vi "Modbus open serial port.vi"(11 "VISA resource name":refnum<visa-resource-name>) -> (0 "Error out":errorcluster, 3 "VISA resource name out":refnum<visa-resource-name>)   [LabVIEW 2020]
doc: "Modbus RTU for Invertek drives. Paul Nathan 18-JUN-2022."
uses:
  <vilib>/Instr/_visa.llb/VISA Open Access Mode.ctl
  Globals/Invertek Drive Params.vi
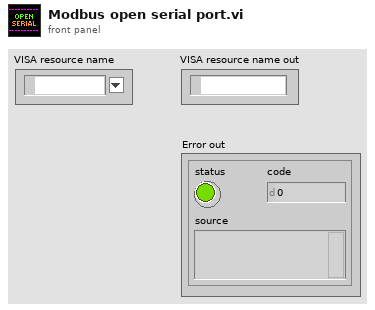
[diagram p1: front panel]
types:
  T1 = typedef "VISA Open Access Mode.ctl" = u32
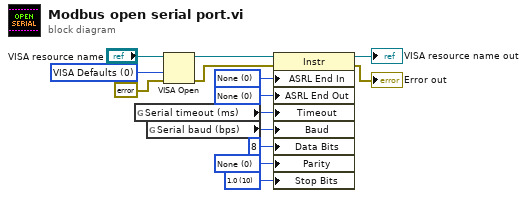
[diagram p0: block diagram]
diagram:
  w3 = u16 10 items=["1.0"=10, "1.5"=15, "2.0"=20] ("Serial Settings:Stop Bits")
  w4 = u16 0 items=["None", "Odd", "Even", "Mark", "Space"] ("Serial Settings:Parity")
  w6 = u16 0 items=["None", "Last Bit", "TermChar", "Break"] ("Serial Settings:End Mode for Writes")
  w11 = u16 0 items=["None", "Last Bit", "TermChar"] ("Serial Settings:End Mode for Reads")
  w14 = T1 0 items=["VISA Defaults"=0, "Exclusive Lock"=1, "Load Configured Settings"=4] ("Access Mode")
  n1 = global read "Invertek Drive Params.vi" "Serial timeout (ms)"() -> (w1:u32)
  n2 = global read "Invertek Drive Params.vi" "Serial baud (bps)"() -> (w2:u32)
  n3 = VISA Open(access mode=w14, error in (no error)=errorcluster {"status"=FALSE, "code"=0, "source"=""}, VISA resource name="VISA resource name") -> (VISA resource name=w8:refnum<visa-resource-name>, error out=w7:errorcluster)  [unwired: 2 in]
  n4 = property class="Instr"(reference=w8, error in=w7, "ASRL End In"=w11, "ASRL End Out"=w6, "Timeout"=w1, "Baud"=w2, "Data Bits"=u16 8 ("Serial Settings:Data Bits"), "Parity"=w4, "Stop Bits"=w3) -> (reference out=→"VISA resource name out":refnum<visa-resource-name>, error out=→"Error out":errorcluster)
